vi "Initialize.vi"(6 "Filter":T1 {"Deny List (ID)" format="%.0x"; "Allow List (ID)" format="%.0x"}, 8 "error in (no error)":errorcluster, 9 "Port Configuration":T2={"Mode"=enum."CAN FD", "Baud Rate"=500000, "Temination On"=TRUE, "Subordinate"=FALSE, "Echo TX"=FALSE, "FD Config"={"FD Baud Rate"=2000000, "ISO Mode"=TRUE, "BRS Enabled"=TRUE}} {"FD Config"."FD Baud Rate" format="%.0p"; "Baud Rate" format="%.0p"}, 10 "Interface":string, 11 "CAN_Logic in":refnum<class "CAN_Logic.lvclass">) -> (0 "error out":errorcluster, 3 "CAN_Logic out":refnum<class "CAN_Logic.lvclass">)   [LabVIEW 2021, in "CAN_Logic.lvclass"]
uses:
  CAN_Logic.lvclass
  typedef/CAN Port Configuration.ctl
  typedef/CAN Mode.ctl
  typedef/FD Config.ctl
  typedef/CAN Filter.ctl
  CAN_Logic.lvclass/CAN_Logic.ctl
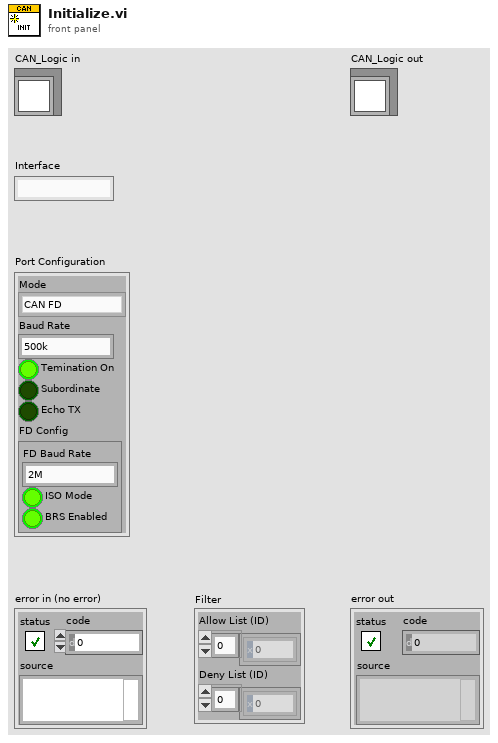
[diagram p1: front panel]
types:
  T1 = typedef "CAN_Logic.lvclass/CAN Filter.ctl" = cluster{"Allow List (ID)":u32[], "Deny List (ID)":u32[]}
  T2 = typedef "CAN_Logic.lvclass/CAN Port Configuration.ctl" = cluster{"Mode":T3, "Baud Rate":u64, "Temination On":bool, "Subordinate":bool, "Echo TX":bool, "FD Config":T4}
  T3 = typedef "CAN_Logic.lvclass/CAN Mode.ctl" = enum16{"CAN 2.0", "CAN FD"}
  T4 = typedef "CAN_Logic.lvclass/FD Config.ctl" = cluster{"FD Baud Rate":u64, "ISO Mode":bool, "BRS Enabled":bool}
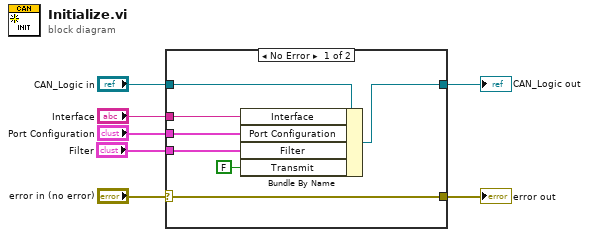
[diagram p0: block diagram]
diagram:
  n1 = case shown="No Error" "error in (no error)" {
    selector: "error in (no error)" -> [w14 w16]
    tunnel: [w14 w16] -> w6
    tunnel: [w10 w15] -> w4
    tunnel: "CAN_Logic in" -> [w13 w15]
    tunnel: "Interface" -> [w12 _]
    tunnel: "Port Configuration" -> [w11 _]
    tunnel: "Filter" -> [w9 _]
    frame No Error {
      n2 = Bundle By Name(cluster=w13, "Interface"=w12, "Port Configuration"=w11, "Filter"=w9, "Transmit"=FALSE) -> (w10:refnum<class "CAN_Logic.lvclass">)
    }
    frame Error {
    }
  }
  "error out" <- w6
  "CAN_Logic out" <- w4
